vi "#66_MAV_MSG_REQUEST_DATA_STREAM_ENCODE.vi"(10 "packet_sequence_in":u8, 11 "REQUEST_DATA_STREAM":T1={"self"={"system_id"=255, "component_id"=190}, "target_system"=1, "target_component"=1, "req_stream_id"=0, "req_message_rate (Hz)"=0, "start_stop"=0}) -> (2 "packet_sequence_out":u8, 3 "mavlink_buffer_out":u8[](array[numeric]))   [LabVIEW 2023]
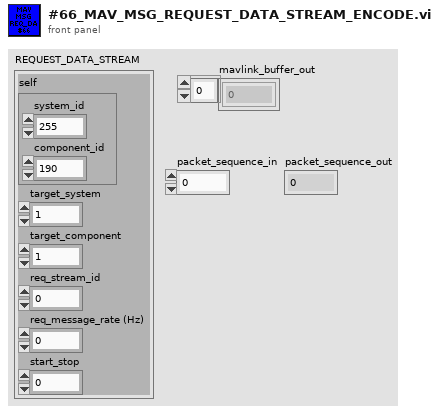
[diagram p1: front panel]
types:
  T1 = cluster{"self":cluster{"system_id":u8, "component_id":u8}, "target_system":u8, "target_component":u8, "req_stream_id":u8, "req_message_rate (Hz)":u16, "start_stop":u8}
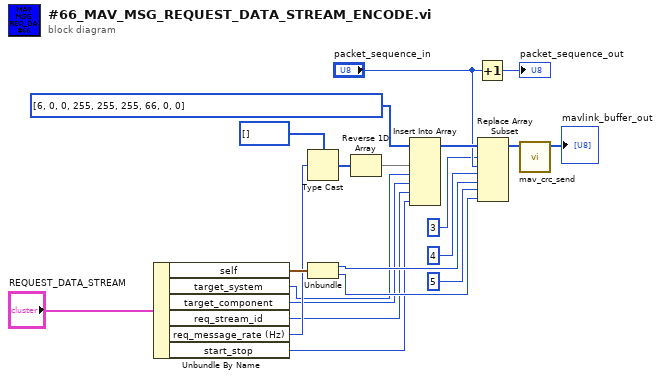
[diagram p0: block diagram]
diagram:
  n1 = Unbundle By Name("REQUEST_DATA_STREAM") -> ("self"=w11:cluster{"system_id":u8, "component_id":u8}, "target_system"=w5:u8, "target_component"=w4:u8, "req_stream_id"=w3:u8, "req_message_rate (Hz)"=w8:u16, "start_stop"=w2:u8)
  n2 = Type Cast(type=u8[] [] ("index"), x=w8) -> (*(type *) &x=w7:u8[])
  n3 = Unbundle(w11) -> ("system_id"=w12:u8, "component_id"=w10:u8)
  n4 = Reverse 1D Array(array=w7) -> (reversed array=w6:u8[])
  n5 = Insert Into Array(array=u8[] [6, 0, 0, 255, 255, 255, 66, 0, 0], new element #1=w6, new element #2=w5, new element #3=w4, new element #4=w3, new element #5=w2) -> (w20:u8[])  [unwired: 1 in]
  n6 = Increment(x="packet_sequence_in") -> (x+1=→"packet_sequence_out":u8)
  n7 = Replace Array Subset(array=w20, new element #1="packet_sequence_in", index #1=3 ("index"), new element #2=w12, index #2=4 ("index"), new element #3=w10, index #3=5 ("index")) -> (w19:u8[])
  n8 = call "mav_crc_send.vi"("Byte In"=w19) -> ("Output Byte"=→"mavlink_buffer_out":u8[])  [unwired: 10 in]
